vi "LVOS Certificates Folder.vi"() -> (1 "cfssl path":path, 3 "Certificates Folder":path)   [LabVIEW 2013]
uses:
  <vilib>/Utility/sysdir.llb/System Directory Type.ctl
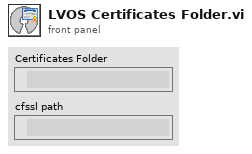
[diagram p1: front panel]
types:
  T1 = typedef "System Directory Type.ctl" = i32
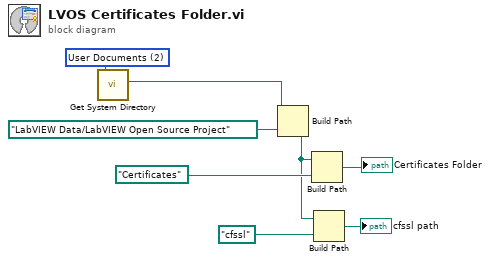
[diagram p0: block diagram]
diagram:
  w6 = T1 2 items=["User Home"=0, "User Desktop"=1, "User Documents"=2, "User Application Data"=3, "User Preferences"=4, "User Temporary"=5, "Public Documents"=6, "Public Application Data"=7, "Public Preferences"=8, "Public Cache"=13, "System Core Libraries"=9, "System Installed Libraries"=10, "Application Files"=11, "Boot Volume Root"=12] ("system directory type")
  n1 = call <vilib>:"Get System Directory.vi"("system directory type"=w6) -> ("system directory"=w8:path)  [unwired: 10 in]
  n2 = Build Path(base path=w8, name or relative path=path "LabVIEW Data/LabVIEW Open Source Project") -> (appended path=w2:path)
  n3 = Build Path(base path=w2, name or relative path=path "Certificates") -> (appended path=→"Certificates Folder":path)
  n4 = Build Path(base path=w2, name or relative path=path "cfssl") -> (appended path=→"cfssl path":path)
